vi "DM-Lin Haobo.vi"() -> ()   [LabVIEW 2017]
panel:
  in  "?":T1(tab)=enum."介电频谱测试"
  in  "测试频率4":dbl=1000.0
  in  "测试频率3":dbl=1000.0
  in  "测试频率1":dbl=1000.0
  in  "测试频率2":dbl=1000.0
  in  "变温速率":dbl=2.0
  in  "结束温度":dbl=200.0
  in  "开始温度":dbl=-60.0
  in  "功能选择":u16(ring) items=["Cp-D", "Cp-Q", "Cp-G", "Cp-Rp", "Cs-D", "Cs-Q", "Cs-Rs", "Lp-D", "Lp-Q", "Lp-G", "Lp-Rp", "Lp-Rdc", "Ls-D", "Ls-Q", "Ls-Rs", "Ls-Rdc", "R-X", "Z-thd", "Z-thr", "G-B", "Y-thd", "Y-thr", "Vdc-Idc"]
  in  "低温":bool
  in  "TCC趋势":bool
  out "残差（损耗）":dbl=100000.0
  out "残差（电容）":dbl=3.0
  in  "LT拟合":u16(ring) items=["多项式", "高斯分布"]
  in  "CT拟合":u16(ring) items=["多项式", "高斯分布", "文献的公式"]
  in  "低温 2":bool
  out "TCC(ppm/℃)":dbl
  in  "表格（L）路径：":path=path "C:/Users/Scrooge/Desktop/CL_LT.xls"
  in  "文本（L）路径：":path=path "C:/Users/Scrooge/Desktop/CL_LT.txt"
  out "LT_LT":cluster{dbl[], dbl[]}(graph)={[50.95, 50.95], [0.0151538, 0.0149556]}
  out "CT_LT":cluster{dbl[], dbl[]}(graph)={[50.95, 50.95], [6.54211e-10, 6.56813e-10]}
  in  "表格（R）路径：":path=path "C:/Users/Scrooge/Desktop/CT_RT.xls"
  in  "文本（R）路径：":path=path "C:/Users/Scrooge/Desktop/CT_RT.txt"
  in  "测试时长（s）":dbl
  in  "测试频率（Hz）":dbl
  in  "开始测量":bool
  out "LT_RT":cluster{dbl[], dbl[]}(graph)
  out "CT_RT":cluster{dbl[], dbl[]}(graph)
  out "?":cluster{dbl[], dbl[]}(graph)={[-5.0, -4.5, -4.0, -3.5, -3.0, -2.5, -2.0, -1.5, -1.0, -0.5, 0.0, 0.5, 1.0, 1.5, 2.0, 2.5, 3.0, 3.5, 4.0, 4.5, 5.0, 5.0, 4.5, 4.0], [0.500691, 0.0469761, 0.379431, 0.495874, 0.487151, 0.476265, 0.495886, 0.531751, 0.471661, 0.519222, 0.521993, 0.503018, 0.492567, 0.515073, 0.507819, 0.532721, 0.517626, 0.519501, 0.453623, 0.435659, 0.488314, 0.175289, 0.0581771, 0.0726732]}
  out "?":cluster{dbl[], dbl[]}(graph)={[-5.0, -4.5, -4.0, -3.5, -3.0, -2.5, -2.0, -1.5, -1.0, -0.5, 0.0, 0.5, 1.0, 1.5, 2.0, 2.5, 3.0, 3.5, 4.0, 4.5, 5.0, 5.0, 4.5, 4.0], [-2.02996e-14, -1.53002e-14, -1.24858e-14, -1.27389e-14, -1.22856e-14, -1.3154e-14, -1.26241e-14, -1.25456e-14, -1.26669e-14, -1.291e-14, -1.26131e-14, -1.30559e-14, -1.2444e-14, -1.26388e-14, -1.22714e-14, -1.28488e-14, -1.30514e-14, -1.28353e-14, -1.3487e-14, -1.35321e-14, -1.2498e-14, -1.39281e-14, -1.68177e-14, -1.62818e-14]}
  in  "文本（BI）路径：":path=path "C:/Users/shipeng/Desktop/BIAS Dielectric measurement Log"
  in  "起始偏压":dbl[][](array[numeric])=[[-5.0, 5.0, 21.0], [5.0, -5.0, 21.0], [-5.0, 0.0, 10.0]]
  in  "偏压":bool
  in  "表格（BI）路径：":path=path "C:/Users/shipeng/Desktop/BIAS Dielectric measurement Log"
  in  "时间间隔(s)":dbl=2.0
  in  "开始频率":dbl[](array[numeric])=[10.0, 10000.0, 100.0]
  in  "频谱":bool
  in  "Scanning Mode":u16(ring)=1 items=["Linear", "Log"]
  in  "文本（SP）路径：":path=path "C:/Users/Scrooge/Desktop/SP.txt"
  out "?":cluster{dbl[], dbl[]}(graph)={[20.0, 22.675383571384522, 25.708651005470756, 29.147676132595485, 33.04673682605462, 37.46737166566934, 42.47935119653383, 48.16177911224783, 54.604340742525736, 61.90871854996752, 70.19019697667008, 79.57948196985141, 90.22476390392299, 102.29405645795312, 115.97784836284757, 131.49210987057194, 149.08170139629277, 169.0242381317775, 191.63447162495464, 217.26925747977248, 246.33318758118733, 279.28497573826183, 316.6446975294954, 359.00199861631705, 407.0254010759322, 461.4728546346695, 523.2036993311451, 593.1922284150527, 672.5430655437831, 762.5085989740041, 864.5087479107281, 980.1533729846564, 1111.2676845606702, 1259.921049894877, 1428.4596538013916, 1619.5435283096847, 1836.1885357487772, 2081.8139678741213, 2360.296512290584, 2676.0314379195047, 3034.0019651954212, 3439.8579158570305, 3900.0048836560754, 4421.705333358719, 5013.193223677282, 5683.803963217401, 6444.121750525505, 7306.146623693386, 8283.483856051174, 9391.558687166586, 10647.85977823354, 12072.215234288142, 13687.105549689764, 15518.01841606206, 17593.850992600805, 19947.365987750378, 22615.70875055146, 25640.99353287359, 29070.968175464932, 32959.76770850899, 37368.76876070874, 42367.55826197211, 48035.031728659946, 54460.63846554949, 61745.793337441646, 70005.47739229642, 79370.05259841043, 89987.31933749607, 102024.84912691955, 115672.62938827681, 131146.0620044891, 148689.36299141843, 168579.41694076196, 191130.14706860675, 216697.46984178963, 245684.9123805555, 278549.9812965547, 315811.3834850681, 358057.21283667657, 405954.2320786253, 460258.39624048397, 521826.78383516293, 591631.1240642137, 670773.1335462716, 760501.904627062, 862233.6197093561, 977573.9027526472, 1108343.1607145814, 1256605.3148961905, 1424700.3756555775, 1615281.374614292, 1831356.2372546163, 2076335.256779795, 2354084.9185135514, 2668988.924345313, 3026017.3803653475, 3430805.2396730217, 3889741.2384150787, 4410068.728724708, 5000000.000000043], [106196000.0, 92409900.0, 81785700.0, 73412700.0, 64489800.0, 57461600.0, 50488800.0, 43921400.0, 38435000.0, 34246700.0, 30339600.0, 26557900.0, 23615000.0, 20839100.0, 18326800.0, 16247600.0, 14299300.0, 12599900.0, 11076900.0, 9796620.0, 8640500.0, 7619490.0, 6707090.0, 5922820.0, 5224210.0, 4612170.0, 4065330.0, 3585910.0, 3159420.0, 2786990.0, 2458510.0, 2169980.0, 1914220.0, 1687870.0, 1489290.0, 1312820.0, 1158360.0, 1021520.0, 901184.0, 794774.0, 700688.0, 618030.0, 545151.0, 480780.0, 424064.0, 374013.0, 329921.0, 290997.0, 256820.0, 226380.0, 199671.0, 176131.0, 155324.0, 137024.0, 120843.0, 106591.0, 94025.6, 82911.0, 73148.6, 64507.3, 56898.9, 50186.7, 44265.8, 39042.2, 34436.3, 30373.6, 26787.8, 23625.0, 20844.2, 18379.7, 16209.0, 14295.6, 12607.4, 11117.7, 9803.59, 8652.08, 7630.04, 6728.0, 5932.48, 5229.76, 4609.8, 4062.43, 3579.4, 3163.33, 2787.36, 2455.53, 2162.54, 1904.44, 1676.44, 1474.35, 1299.56, 1140.07, 995.777, 823.897, 705.8, 596.582, 494.824, 397.785, 377.206, 304.016]}
  out "?":cluster{dbl[], dbl[]}(graph)={[20.0, 22.675383571384522, 25.708651005470756, 29.147676132595485, 33.04673682605462, 37.46737166566934, 42.47935119653383, 48.16177911224783, 54.604340742525736, 61.90871854996752, 70.19019697667008, 79.57948196985141, 90.22476390392299, 102.29405645795312, 115.97784836284757, 131.49210987057194, 149.08170139629277, 169.0242381317775, 191.63447162495464, 217.26925747977248, 246.33318758118733, 279.28497573826183, 316.6446975294954, 359.00199861631705, 407.0254010759322, 461.4728546346695, 523.2036993311451, 593.1922284150527, 672.5430655437831, 762.5085989740041, 864.5087479107281, 980.1533729846564, 1111.2676845606702, 1259.921049894877, 1428.4596538013916, 1619.5435283096847, 1836.1885357487772, 2081.8139678741213, 2360.296512290584, 2676.0314379195047, 3034.0019651954212, 3439.8579158570305, 3900.0048836560754, 4421.705333358719, 5013.193223677282, 5683.803963217401, 6444.121750525505, 7306.146623693386, 8283.483856051174, 9391.558687166586, 10647.85977823354, 12072.215234288142, 13687.105549689764, 15518.01841606206, 17593.850992600805, 19947.365987750378, 22615.70875055146, 25640.99353287359, 29070.968175464932, 32959.76770850899, 37368.76876070874, 42367.55826197211, 48035.031728659946, 54460.63846554949, 61745.793337441646, 70005.47739229642, 79370.05259841043, 89987.31933749607, 102024.84912691955, 115672.62938827681, 131146.0620044891, 148689.36299141843, 168579.41694076196, 191130.14706860675, 216697.46984178963, 245684.9123805555, 278549.9812965547, 315811.3834850681, 358057.21283667657, 405954.2320786253, 460258.39624048397, 521826.78383516293, 591631.1240642137, 670773.1335462716, 760501.904627062, 862233.6197093561, 977573.9027526472, 1108343.1607145814, 1256605.3148961905, 1424700.3756555775, 1615281.374614292, 1831356.2372546163, 2076335.256779795, 2354084.9185135514, 2668988.924345313, 3026017.3803653475, 3430805.2396730217, 3889741.2384150787, 4410068.728724708, 5000000.000000043], [106196000.0, 92409900.0, 81785700.0, 73412700.0, 64489800.0, 57461600.0, 50488800.0, 43921400.0, 38435000.0, 34246700.0, 30339600.0, 26557900.0, 23615000.0, 20839100.0, 18326800.0, 16247600.0, 14299300.0, 12599900.0, 11076900.0, 9796620.0, 8640500.0, 7619490.0, 6707090.0, 5922820.0, 5224210.0, 4612170.0, 4065330.0, 3585910.0, 3159420.0, 2786990.0, 2458510.0, 2169980.0, 1914220.0, 1687870.0, 1489290.0, 1312820.0, 1158360.0, 1021520.0, 901184.0, 794774.0, 700688.0, 618030.0, 545151.0, 480780.0, 424064.0, 374013.0, 329921.0, 290997.0, 256820.0, 226380.0, 199671.0, 176131.0, 155324.0, 137024.0, 120843.0, 106591.0, 94025.6, 82911.0, 73148.6, 64507.3, 56898.9, 50186.7, 44265.8, 39042.2, 34436.3, 30373.6, 26787.8, 23625.0, 20844.2, 18379.7, 16209.0, 14295.6, 12607.4, 11117.7, 9803.59, 8652.08, 7630.04, 6728.0, 5932.48, 5229.76, 4609.8, 4062.43, 3579.4, 3163.33, 2787.36, 2455.53, 2162.54, 1904.44, 1676.44, 1474.35, 1299.56, 1140.07, 995.777, 823.897, 705.8, 596.582, 494.824, 397.785, 377.206, 304.016]}
  in  "表格（SP）路径：":path=path "C:/Users/Scrooge/Desktop/SP.xls"
  in  "使用6517B":bool
  in  "样本厚度(mm)":dbl
  in  "样本直径(mm)":dbl
  in  "电压(V)":dbl
  in  "测试时间":dbl
  in  "绝缘":bool
  out "?":cluster{dbl[], dbl[]}(graph)={[0.201, 1.192, 2.172, 3.151, 4.129, 5.107, 6.086, 7.064, 8.042, 9.021, 10.0, 10.978, 11.957, 12.935, 13.913, 14.891, 15.87, 16.849, 17.827, 18.807, 19.789, 20.767, 21.746, 22.724, 23.702, 24.68, 25.659, 26.637, 27.616, 28.595, 29.558, 30.536, 31.514, 32.493, 33.472, 34.45, 35.43, 36.408, 37.386, 38.365, 39.344, 40.339], [-1675.86, -1675.85, -1676.0, -1676.13, -1676.17, -1676.27, -1677.48, -1675.99, -1676.43, -1681.46, -1676.29, -1676.08, -1676.1, -1676.02, -1675.83, -1675.8, -1675.82, -1675.56, -1675.6, -1675.32, -1675.21, -1674.89, -1674.7, -1674.46, -1673.99, -1673.55, -1673.08, -1672.36, -1671.64, -1670.87, -1670.26, -1669.55, -1668.7, -1667.65, -1666.77, -1665.8, -1664.61, -1663.41, -1662.55, -1661.04, -1659.56, -1657.68]}
  out "?":cluster{dbl[], dbl[]}(graph)={[0.201, 1.192, 2.172, 3.151, 4.129, 5.107, 6.086, 7.064, 8.042, 9.021, 10.0, 10.978, 11.957, 12.935, 13.913, 14.891, 15.87, 16.849, 17.827, 18.807, 19.789, 20.767, 21.746, 22.724, 23.702, 24.68, 25.659, 26.637, 27.616, 28.595, 29.558, 30.536, 31.514, 32.493, 33.472, 34.45, 35.43, 36.408, 37.386, 38.365, 39.344, 40.339], [9665.96, 9670.54, 9661.83, 9662.16, 9663.16, 9703.15, 9737.63, 9698.46, 9692.46, 9806.7, 9560.83, 9481.19, 9418.37, 9320.17, 9268.16, 9226.14, 9160.9, 9088.06, 9034.83, 8929.32, 8815.93, 8688.35, 8579.32, 8438.3, 8233.36, 8027.73, 7834.66, 7575.86, 7313.56, 7056.58, 6882.85, 6681.73, 6437.13, 6185.99, 5948.9, 5748.35, 5507.66, 5280.44, 5128.46, 4857.69, 4620.19, 4342.91]}
  in  "文本（IN）路径：":path=path "C:/Users/Scrooge/Desktop/IN.txt"
  in  "表格（IN）路径：":path=path "C:/Users/Scrooge/Desktop/IN.xls"
  out "样品温度":dbl
  out "设定温度":dbl
  out "炉丝温度":dbl
  in  "测试温度":dbl
  out "当前频率":dbl
  in  "开始测量":bool
  out "?":cluster{dbl[], dbl[]}(graph)={[4.76578, 4.95183, 5.2639, 5.45631, 5.68923, 5.96482, 6.29877, 6.6422, 6.96399, 7.34085, 7.76822, 8.17855, 8.63274, 9.15865, 9.79553, 10.5502, 11.0706, 11.9952, 12.9319, 13.9265, 15.0197, 16.3568, 17.7532, 19.3246, 21.0927, 23.0242, 25.0623, 27.5307, 29.9738, 33.2177, 36.5272, 40.3473, 44.6699, 49.3322, 54.7469, 60.6627, 67.4071, 74.9786, 83.5253, 93.1379, 104.03, 116.389, 130.429, 145.987, 163.909, 183.98, 206.64, 232.188, 258.147, 291.919, 335.859, 374.84, 414.539, 465.991, 532.048, 602.949, 689.134, 773.249, 870.102, 985.903, 1123.13, 1275.36, 1451.73, 1641.81, 1865.44, 2115.4, 2399.17, 2720.93, 3089.67, 3508.29, 3980.83, 4515.29, 5118.64, 5799.71, 6605.19, 7472.24, 8449.86, 9551.85, 10779.4, 12163.7, 13702.2, 15433.1, 17391.2, 19544.4, 21947.6, 24613.1, 27562.8, 30840.7, 34475.5, 38529.5, 42968.4, 47826.9, 53184.8, 59163.2, 65651.7, 72759.1, 80688.8, 89228.1, 98569.2, 109036.0, 119923.0, 132208.0, 145083.0, 160265.0, 175774.0, 193159.0, 211401.0, 233068.0, 252305.0, 278064.0, 302611.0, 331752.0, 363430.0, 397628.0, 432832.0, 469048.0, 511668.0, 554491.0, 605253.0, 655000.0, 713841.0, 767324.0, 831011.0, 905837.0, 971237.0, 1047330.0, 1135590.0, 1242550.0, 1324860.0, 1419260.0, 1528060.0, 1657260.0, 1657060.0, 1657050.0, 1656970.0], [-83.8388, -94.0695, -105.065, -116.633, -129.293, -142.98, -157.704, -173.594, -190.768, -209.471, -229.697, -251.716, -275.643, -301.645, -329.901, -360.642, -393.025, -429.595, -469.363, -512.712, -559.92, -611.338, -667.345, -728.401, -794.926, -867.436, -946.529, -1032.74, -1127.27, -1229.64, -1341.14, -1462.94, -1595.66, -1740.3, -1897.85, -2069.31, -2256.7, -2460.9, -2683.52, -2926.12, -3190.55, -3478.51, -3792.28, -4134.43, -4507.09, -4913.34, -5355.9, -5837.88, -6361.18, -6940.5, -7557.26, -8227.75, -8966.19, -9776.49, -10656.2, -11603.4, -12634.8, -13758.9, -14987.4, -16326.3, -17778.6, -19343.5, -21058.8, -22912.4, -24935.1, -27125.7, -29507.3, -32090.3, -34889.3, -37930.7, -41217.4, -44779.7, -48622.7, -52802.5, -57377.3, -62244.1, -67524.9, -73242.8, -79372.7, -86027.9, -93155.5, -100863.0, -109184.0, -118105.0, -127741.0, -138062.0, -149118.0, -160966.0, -173746.0, -187598.0, -202286.0, -217928.0, -234691.0, -252890.0, -272113.0, -292631.0, -314916.0, -338309.0, -363290.0, -390625.0, -418327.0, -449446.0, -481377.0, -517085.0, -552683.0, -591702.0, -631650.0, -677951.0, -720582.0, -773764.0, -824284.0, -882606.0, -943903.0, -1007950.0, -1073950.0, -1140070.0, -1216170.0, -1291290.0, -1378160.0, -1461580.0, -1558420.0, -1642670.0, -1743870.0, -1859760.0, -1958990.0, -2071380.0, -2200810.0, -2350980.0, -2464640.0, -2593280.0, -2739320.0, -2906600.0, -2906310.0, -2905990.0, -2905750.0]}
  in  "表格（CC）路径：":path=path "C:/Users/Scrooge/Desktop/CC.xls"
  in  "文本（CC）路径：":path=path "C:/Users/Scrooge/Desktop/CC.txt"
  in  "开始频率":dbl[](array[numeric])=[20.0, 5000000.0, 100.0]
  in  "扫描模式":u16(ring)=1 items=["Linear", "Log"]
  in  "极化开始":bool
  out "剩余时间":dbl
  out "极化状态":bool
  out "当前温度":dbl
  in  "结束冷却":bool
  in  "结束温度（℃）":dbl
  in  "变温速率（℃/min）":dbl
  in  "极化时间":dbl
  in  "极化电压（V）":dbl
  in  "极化温度（℃）":dbl
  out "当前去极化电流":dbl
  in  "文本（TSDC）路径：":path=path "C:/Users/Scrooge/Desktop/TSDC.txt"
  out "?":cluster{dbl[], dbl[]}(graph)
  in  "温度":bool
  in  "变温速率1":dbl=3.0
  in  "目标温度":dbl=255.0
  out "TE":cluster{dbl[], dbl[]}(graph)={[0.0, 2.0, 4.0, 6.001, 8.001, 10.001, 12.001, 14.002, 16.002, 18.002, 20.003, 22.003, 24.003, 26.003, 28.003, 30.003, 32.003, 34.003, 36.003, 38.003, 40.003, 42.004, 44.004, 46.004, 48.005, 50.006, 52.006, 54.006, 56.006, 58.007, 60.007, 62.007, 64.007, 66.007, 68.007, 70.007, 72.007, 74.008, 76.008, 78.008, 80.008, 82.008, 84.008, 86.008, 88.008, 90.008, 92.008, 94.008, 96.008, 98.008, 100.009, 102.01, 104.01, 106.01, 108.01, 110.01, 112.01, 114.01, 116.01, 118.01, 120.01, 122.01, 124.011, 126.012, 128.012, 130.013, 132.013, 134.014, 136.014, 138.014, 140.014, 142.014, 144.014, 146.014, 148.014, 150.014, 152.015, 154.015, 156.016, 158.016, 160.016, 162.016, 164.016, 166.016, 168.016, 170.016, 172.017, 174.017, 176.018, 178.018, 180.019, 182.019, 184.019, 186.019, 188.02, 190.02, 192.02, 194.02, 196.021, 198.021, 200.021, 202.022, 204.022, 206.022, 208.022, 210.023, 212.023, 214.023, 216.023, 218.023, 220.023, 222.024, 224.025, 226.025, 228.026, 230.026, 232.026, 234.026, 236.026, 238.026, 240.026, 242.026, 244.027, 246.028, 248.028, 250.028, 252.028, 254.028, 256.028, 258.028, 260.028, 262.028, 264.028, 266.028, 268.028, 270.029, 272.029, 274.029, 276.029, 278.029, 280.029, 282.03, 284.03, 286.03, 288.031, 290.031, 292.031, 294.031, 296.031, 298.031, 300.031, 302.032, 304.032, 306.032, 308.032, 310.032, 312.032, 314.032, 316.615, 318.616, 320.616, 322.616, 324.616, 326.616, 328.616, 330.616, 332.616, 334.617, 336.617, 338.617, 340.617, 342.617, 344.617, 346.617, 348.617, 350.617, 352.617, 354.618, 356.618, 358.618, 360.618, 362.618, 364.619, 366.619, 368.619, 370.62, 372.62, 374.62, 376.621, 378.621, 380.622, 382.622, 384.622, 386.622, 388.622, 390.623, 392.623, 394.623, 396.623, 398.623, 400.624, 402.624, 404.624, 406.624, 408.624, 410.625, 412.625, 414.625, 416.625, 418.625, 420.625, 422.625, 424.626, 426.626, 428.626, 430.627, 432.627, 434.627, 436.627, 438.628, 440.628, 442.628, 444.628, 446.628, 448.628, 450.628, 452.628, 454.629, 456.629, 458.63, 460.63, 462.63, 464.63, 466.63, 468.63, 470.63, 472.63, 474.63, 476.63, 478.631, 480.631, 482.632, 484.632, 486.632, 488.632, 490.632, 492.633, 494.633, 496.633, 498.633, 500.633, 502.633, 504.633, 506.633, 508.633, 510.633, 512.633, 514.633, 516.633, 518.633, 520.633, 522.633, 524.633, 526.633, 528.633, 530.634, 532.634, 534.634, 536.634, 538.634, 540.634, 542.635, 544.635, 546.635, 548.635, 550.635, 552.635, 554.636, 581.094, 583.094, 585.095, 587.095, 589.095, 591.095, 593.096, 595.097, 597.097, 599.097, 601.097, 603.097, 605.097, 607.097, 609.097, 611.098, 613.099, 615.099, 617.099, 621.973, 623.973, 625.973, 627.973, 629.973, 631.973, 633.973, 635.973, 637.973, 639.973, 641.973, 643.974, 648.231, 650.231, 652.231, 654.231, 656.231, 658.231, 660.231, 662.231, 664.231, 666.231, 668.231], [50.0, 50.0, 49.96, 49.910000000000004, 49.84, 49.77, 49.72, 49.68, 49.63, 49.47, 49.46, 49.51, 49.57, 49.64, 49.77, 49.85, 49.77, 49.800000000000004, 49.88, 50.0, 50.13, 50.29, 50.370000000000005, 50.5, 50.620000000000005, 50.74, 50.92, 50.84, 50.910000000000004, 50.980000000000004, 51.06, 51.14, 51.31, 51.43, 51.550000000000004, 51.68, 51.76, 51.88, 51.83, 51.910000000000004, 51.99, 52.120000000000005, 52.2, 52.28, 52.36, 52.480000000000004, 52.61, 52.78, 52.86, 52.75, 52.81, 52.88, 52.96, 53.09, 53.21, 53.33, 53.42, 53.54, 53.620000000000005, 53.71, 53.620000000000005, 53.65, 53.78, 53.86, 53.93, 54.02, 54.1, 54.18, 54.27, 54.43, 54.550000000000004, 54.46, 54.54, 54.620000000000005, 54.75, 54.88, 55.04, 55.21, 55.33, 55.45, 55.58, 55.75, 55.69, 55.78, 55.86, 55.980000000000004, 56.07, 56.24, 56.36, 56.49, 56.61, 56.74, 56.78, 56.79, 56.88, 57.0, 57.08, 57.17, 57.25, 57.410000000000004, 57.54, 57.660000000000004, 57.78, 57.870000000000005, 57.78, 57.86, 57.99, 58.11, 58.230000000000004, 58.31, 58.44, 58.52, 58.69, 58.85, 58.89, 58.85, 58.93, 59.050000000000004, 59.18, 59.34, 59.42, 59.550000000000004, 59.67, 59.79, 59.96, 59.99, 60.01, 60.09, 60.18, 60.300000000000004, 60.47, 60.59, 60.71, 60.84, 60.96, 61.08, 61.14, 61.13, 61.21, 61.34, 61.42, 61.5, 61.67, 61.79, 61.910000000000004, 62.04, 62.160000000000004, 62.190000000000005, 62.17, 62.29, 62.410000000000004, 62.5, 62.620000000000005, 62.7, 62.83, 62.96, 63.120000000000005, 63.13, 63.120000000000005, 63.24, 63.32, 63.52, 63.65, 63.77, 63.85, 63.980000000000004, 64.06, 64.26, 64.29, 64.29, 64.37, 64.5, 64.62, 64.78, 64.91, 65.03, 65.15, 65.28, 65.36, 65.48, 65.49, 65.57000000000001, 65.65, 65.78, 65.86, 66.03, 66.16, 66.28, 66.36, 66.53, 66.44, 66.48, 66.61, 66.73, 66.85, 66.94, 67.02, 67.14, 67.31, 67.43, 67.55, 67.5, 67.55, 67.63, 67.8, 67.92, 68.0, 68.17, 68.25, 68.37, 68.55, 68.67, 68.65, 68.65, 68.73, 68.85000000000001, 69.02, 69.18, 69.3, 69.43, 69.55, 69.67, 69.84, 69.8, 69.84, 69.93, 70.01, 70.13, 70.3, 70.42, 70.54, 70.67, 70.79, 70.91, 70.87, 70.95, 71.03, 71.12, 71.2, 71.32000000000001, 71.45, 71.61, 71.73, 71.86, 71.98, 71.88, 71.94, 72.10000000000001, 72.18, 72.31, 72.43, 72.5, 72.67, 72.83, 72.95, 73.08, 73.05, 73.07000000000001, 73.16, 73.29, 73.41, 73.54, 73.7, 73.82000000000001, 73.91, 74.08, 74.2, 74.16, 74.23, 74.29, 74.42, 74.55, 74.67, 74.8, 74.92, 75.04, 75.17, 76.37, 76.4, 76.53, 76.65, 76.73, 76.82000000000001, 76.98, 77.15, 77.28, 77.4, 77.47, 77.41, 77.49, 77.62, 77.75, 77.87, 77.99, 78.08, 78.2, 78.56, 78.48, 78.51, 78.56, 78.63, 78.71000000000001, 78.79, 78.92, 79.04, 79.12, 79.25, 79.33, 79.25, 79.26, 79.28, 79.33, 79.35000000000001, 79.42, 79.47, 79.52, 79.58, 79.69, 79.53, 79.52]} caption="1"
  in  "远程模式":bool
  out "错误输出":cluster{"状态":bool, "代码":i32, "源":string}={"状态"=FALSE, "代码"=-1950679034, "源"="DM-Lin Haobo.vi中的共享变量<APPEND>\n读取以下共享变量时发生该错误或警告：\n\\\\我的电脑\\Input\\Start_LT\n\\\\10.21.14.98\\Input\\Start_LT"}
  in  "error in (no error)":errorcluster caption="错误输入（无错误）"
  in  "电阻计地址":refnum<visa-resource-name>
  in  "低温地址":refnum<visa-resource-name>
  in  "高温地址 1":refnum<visa-resource-name> caption="高温地址1"
  in  "高温地址 2":refnum<visa-resource-name> caption="高温地址2"
  in  "电容计地址":refnum<visa-resource-name>
  # "参数1-温度"
  # "参数2-温度/TCC"
  # "电容-时间"
  # "损耗-时间"
  # "结束偏压"
  # "步长"
  # "结束频率"
  # "步数"
  # "基本功能"
  # "K6517B功能"
  # "电阻值（TH2826）-时间\n电阻率（K6517B）-时间"
  # "电抗（TH2826）-时间\n电流（K6517B）-时间"
  # "Z'-Z''(R-X)"
  # "操作步骤：\n1.输入数据保存路径\n2.设置极化温度、极化电压、极化时间\n3.点击“极化开始”按钮，等待温度达到极化温度\n4.当极化温度达到设定温度后观察“极化状态”指示灯\n5.若“极化状态”指示灯亮起，则意味着极化电压已正常启动\n6.极化电压启动后观察“剩余时间”，当其为0时极化结束\n7.极化结束后请尽快开启液氮冷却样品\n8.要开始测电流请先在“结束温度”输入框内填入测量结束温度\n9.按下“结束冷却”按钮，极化电压将关闭，TSDC测量开始\n注意：\n1.“变温速率”=极化前升温速=极化后降温速=测电流升温速\n2.开始测电流的三个条件：\n2.1.“结束冷却”按钮被按下\n2.2.“当前温度”低于-20（摄氏度）\n2.3.“剩余时间”为0"
  # "TSDC-温度"
  # "温度-时间"
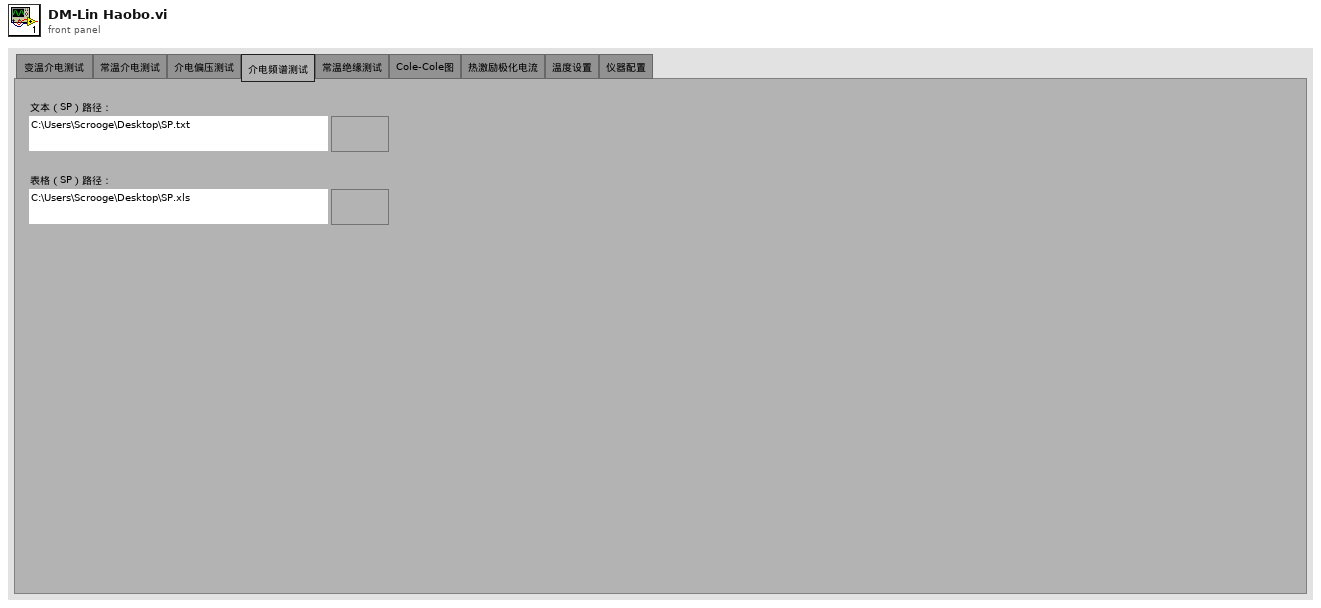
[diagram p1: front panel]
types:
  T1 = enum32{"变温介电测试 ", "常温介电测试", "介电偏压测试", "介电频谱测试", "常温绝缘测试", "Cole-Cole图", "热激励极化电流", "温度设置", "仪器配置"}
  T2 = cluster{"测试频率1":dbl, "测试频率2":dbl, "测试频率3":dbl, "测试频率4":dbl}
  T3 = cluster{"CT_LT":cluster{dbl[], dbl[]}, "LT_LT":cluster{dbl[], dbl[]}}
  T4 = cluster{"电容计地址":refnum<visa-resource-name>, "高温地址 1":refnum<visa-resource-name>, "高温地址 2":refnum<visa-resource-name>}
  T5 = cluster{"开始温度":dbl, "变温速率":dbl, "结束温度":dbl, cluster{"测试频率1":dbl, "测试频率2":dbl, "测试频率3":dbl, "测试频率4":dbl}}
  T6 = cluster{"电容计地址":refnum<visa-resource-name>, "低温地址":refnum<visa-resource-name>}
  T7 = cluster{"电阻计地址":refnum<visa-resource-name>, "电容计地址":refnum<visa-resource-name>, "低温地址":refnum<visa-resource-name>, "高温地址 2":refnum<visa-resource-name>}
  T8 = cluster{"电压(V)":dbl, "样本直径(mm)":dbl, "样本厚度(mm)":dbl}
  T9 = cluster{"Ctrl Reference":refnum<vi>, "当前频率":refnum<vi>, "炉丝温度":refnum<vi>, "设定温度":refnum<vi>, "样品温度":refnum<vi>}
  T10 = cluster{"电阻计地址":refnum<visa-resource-name>, "高温地址 1":refnum<visa-resource-name>, "高温地址 2":refnum<visa-resource-name>}
  T11 = cluster{"变温速率（℃/min）":dbl, "极化温度（℃）":dbl, "极化电压（V）":dbl, "极化时间":dbl}
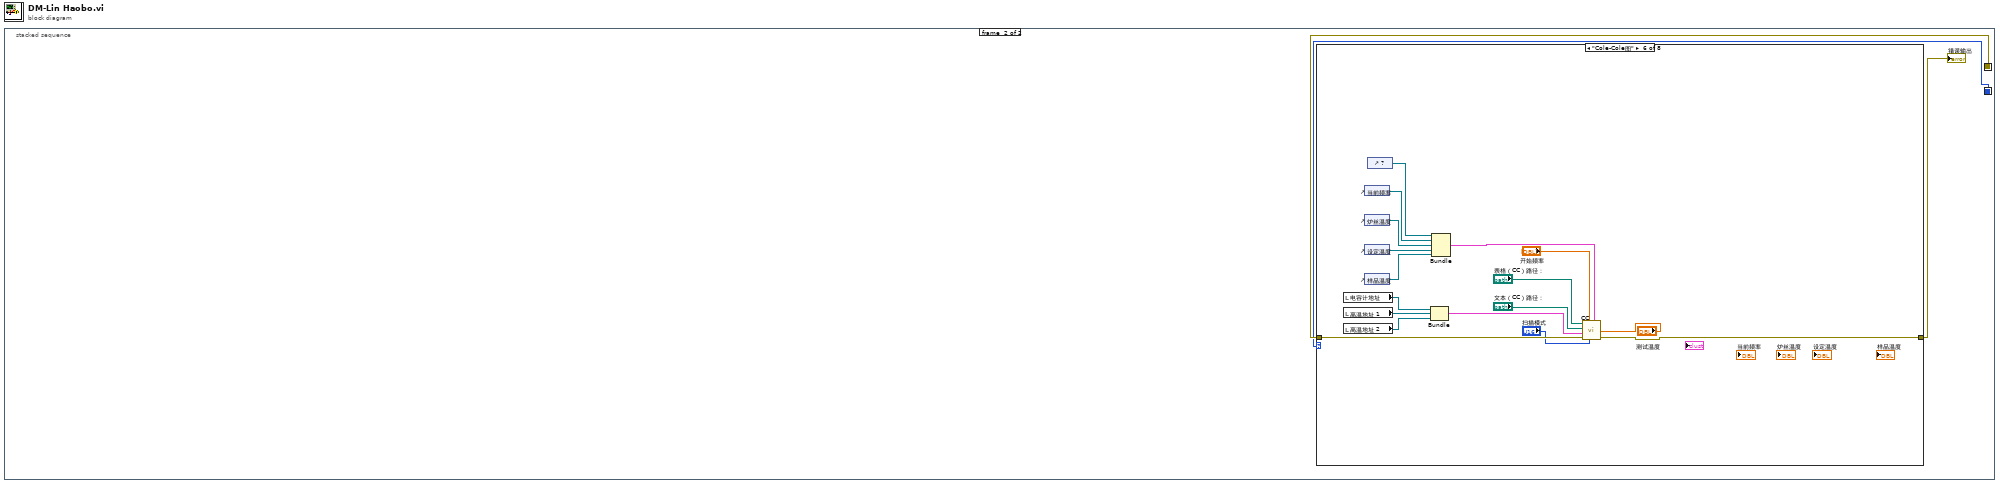
[diagram p0: block diagram]
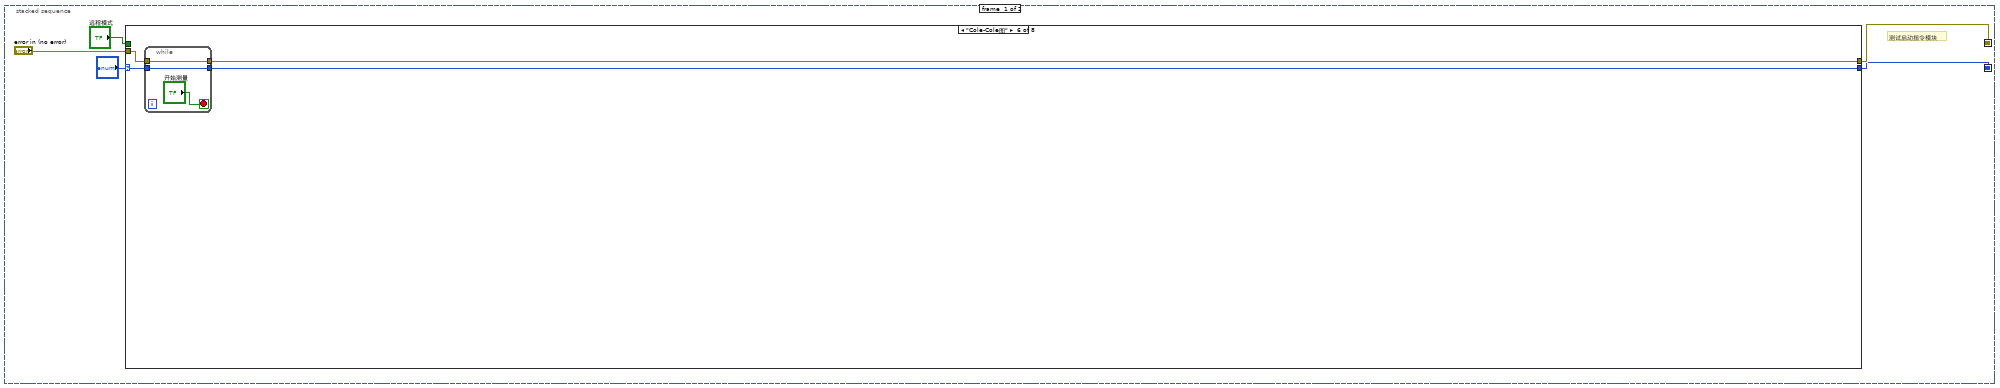
[diagram p2: hidden frame]
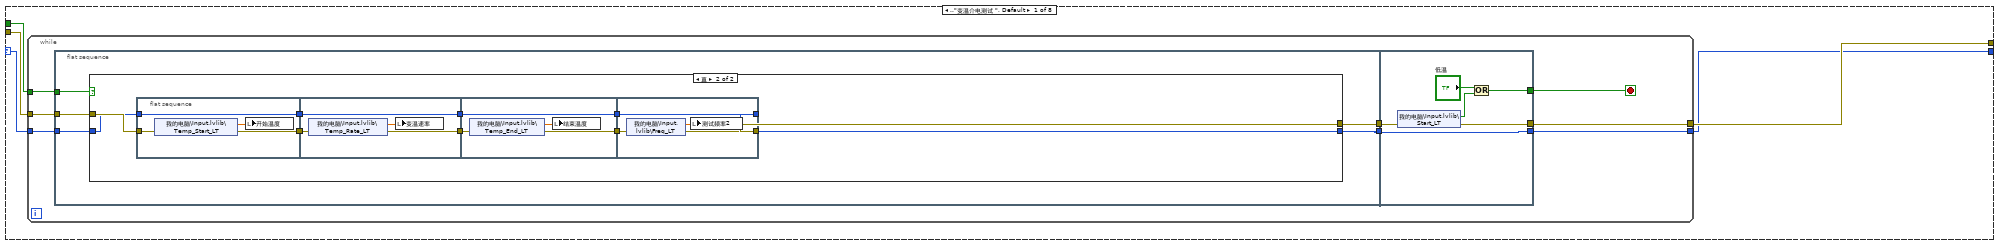
[diagram p3: hidden frame]
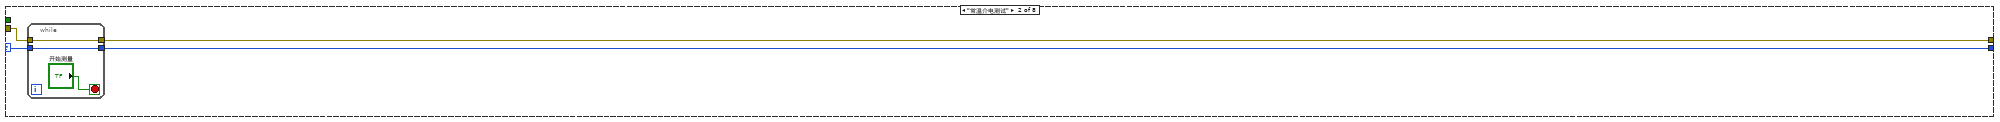
[diagram p5: hidden frame]
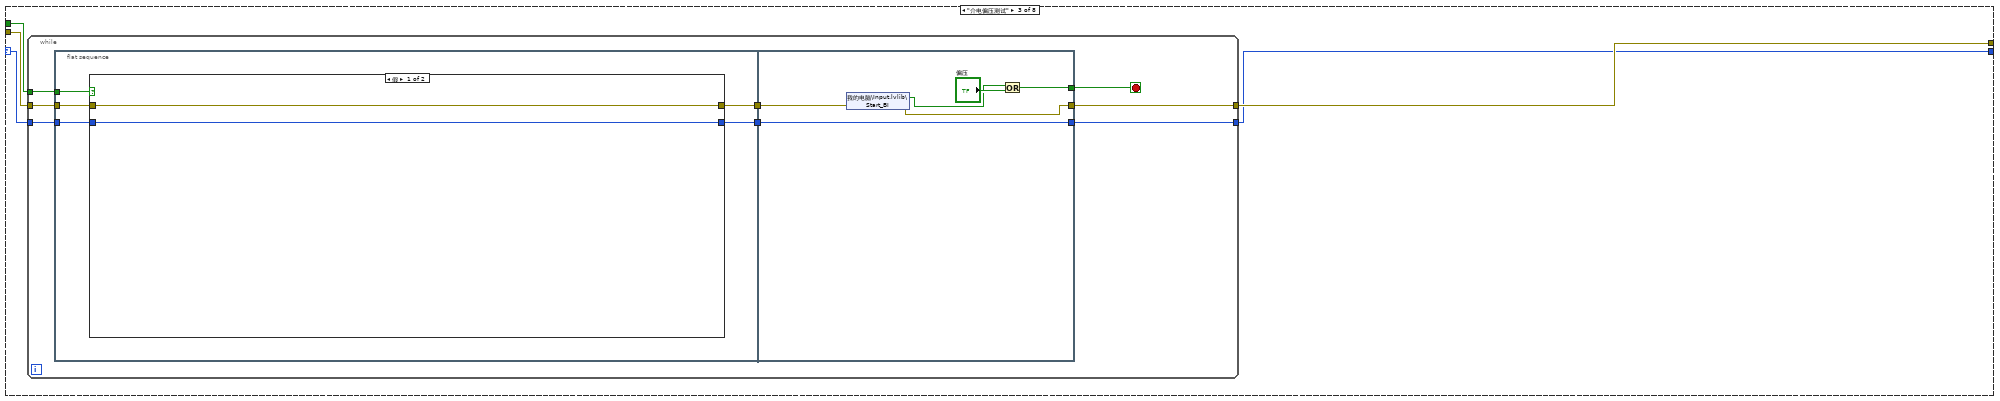
[diagram p6: hidden frame]
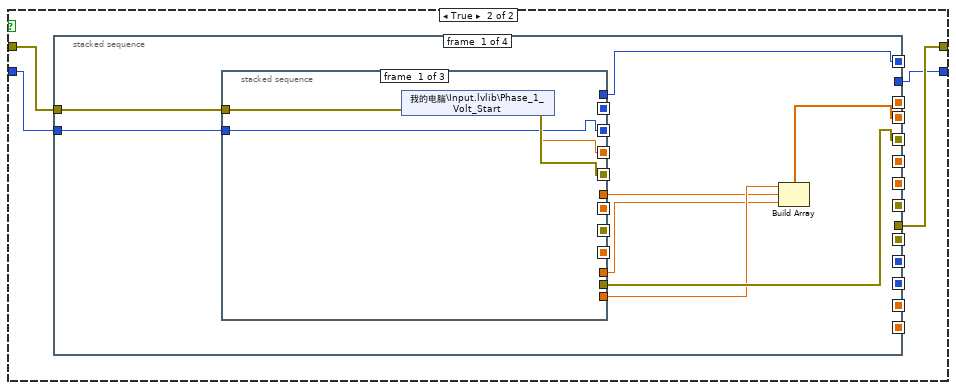
[diagram p7: hidden frame]
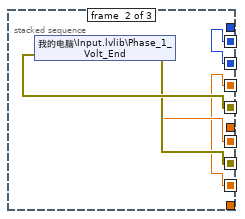
[diagram p8: hidden frame]
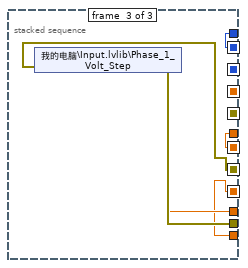
[diagram p9: hidden frame]
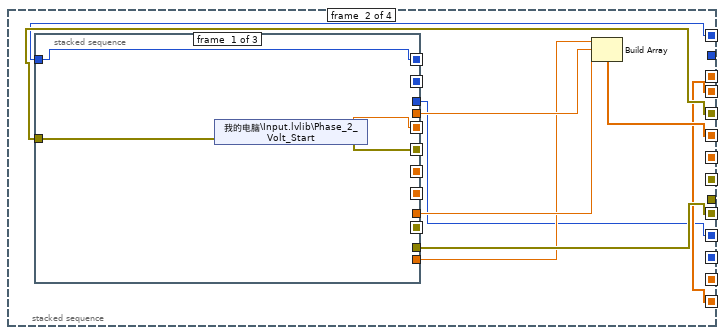
[diagram p10: hidden frame]
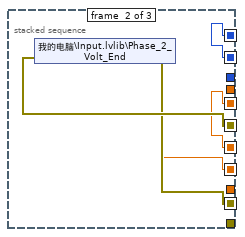
[diagram p11: hidden frame]
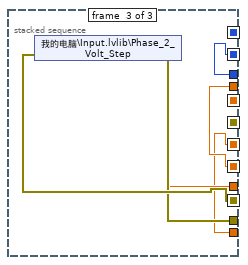
[diagram p12: hidden frame]
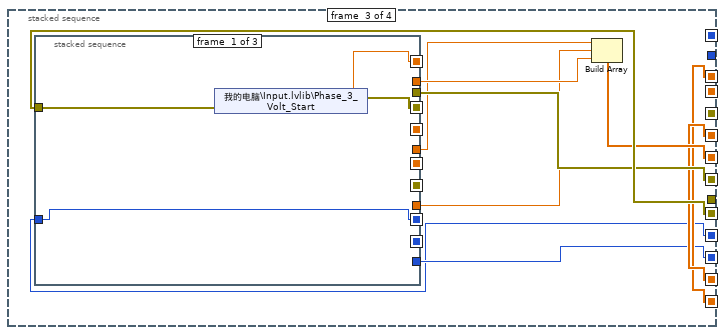
[diagram p13: hidden frame]
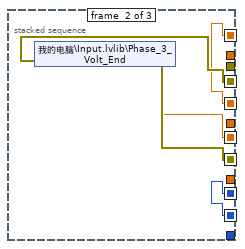
[diagram p14: hidden frame]
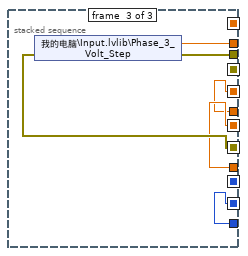
[diagram p15: hidden frame]
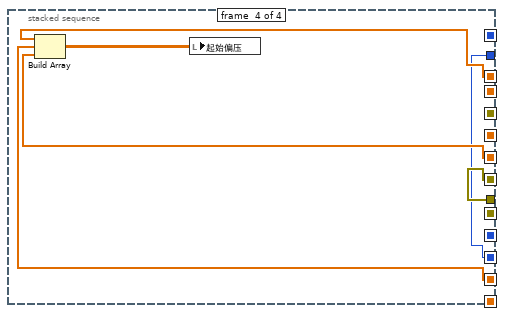
[diagram p16: hidden frame]
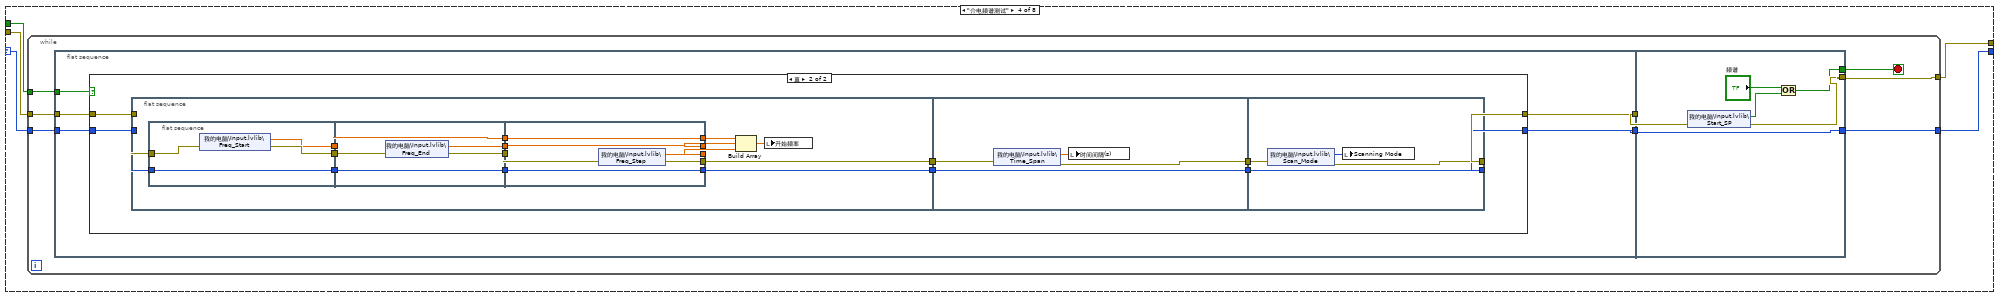
[diagram p17: hidden frame]
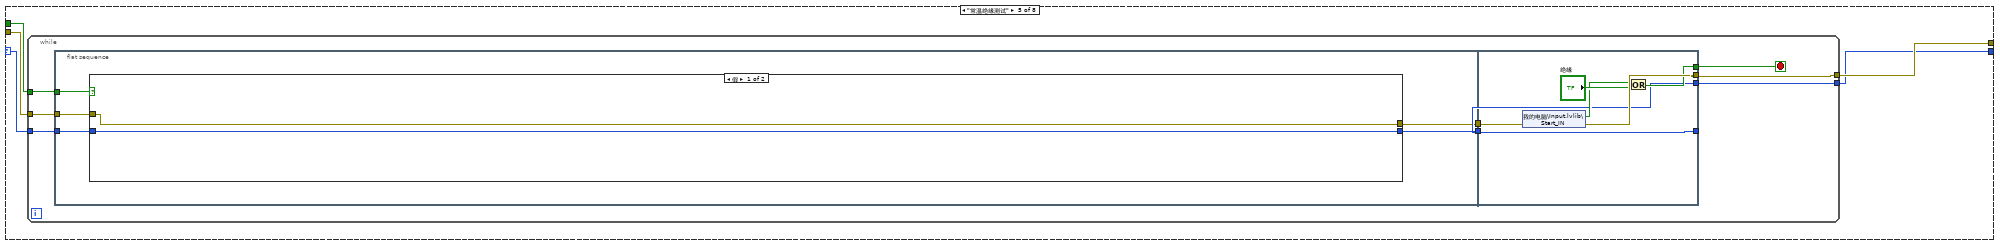
[diagram p19: hidden frame]
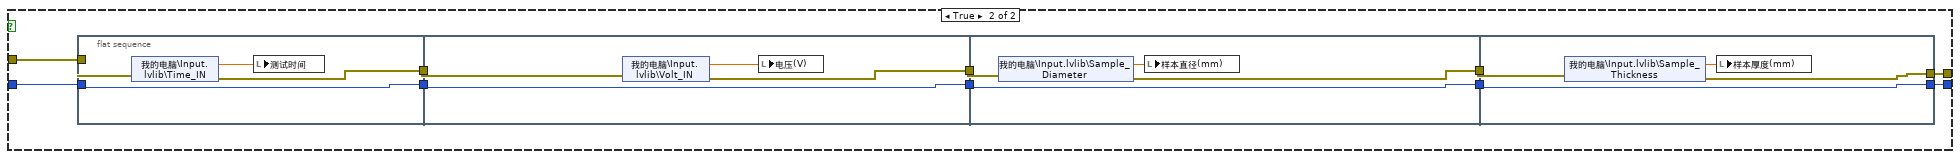
[diagram p20: hidden frame]
diagram:
  n1 = stacked-sequence {
    seq-local: [w1 _] -> [_ w351]
    seq-local: [w5 _] -> [_ w353]
    frame #0 {
      # "测试启动指令模块"
      n2 = case shown="\"Cole-Cole图\"" "?" {
        selector: "?" -> [w6 w59 w66 w173 w246 w300 w305 w312]
        tunnel: [w9 w61 w67 w175 w247 w297 w306 w313] -> w5
        tunnel: "error in (no error)" -> [w10 w60 w69 w177 w249 w298 w307 w315]
        tunnel: "远程模式" -> [w8 _ w68 w176 w248 _ _ w314]
        tunnel: [w7 w58 w65 w174 w245 w299 w304 w311] -> w1
        frame .."变温介电测试 ", Default {
          n3 = while {
            tunnel: w10 -> [w18]
            tunnel: [w17] -> w9
            tunnel: w8 -> [w14]
            tunnel: [w13] -> w7
            tunnel: w6 -> [w11]
            stop <- w16 stop-if-true
            n4 = flat-sequence {
              tunnel: w18 -> [w23]
              tunnel: [w22] -> w15
              tunnel: w14 -> [w21]
              tunnel: [w20] -> w12
              tunnel: w11 -> [w19]
              tunnel: [w57] -> w17
              tunnel: [w56] -> w16
              tunnel: w15 -> [w53]
              tunnel: [w52] -> w13
              tunnel: w12 -> [w52]
              frame #0 {
                n5 = case shown="真" w21 {
                  tunnel: w23 -> [w25 w35]
                  tunnel: [w25 w34] -> w22
                  tunnel: [w24 w30] -> w20
                  tunnel: w19 -> [w24 w26]
                  frame False {
                  }
                  frame True {
                    n6 = flat-sequence {
                      tunnel: w35 -> [w39]
                      tunnel: [w37] -> w33
                      tunnel: [w36] -> w27
                      tunnel: w26 -> [w36]
                      tunnel: w33 -> [w43]
                      tunnel: [w41] -> w32
                      tunnel: [w40] -> w28
                      tunnel: w27 -> [w40]
                      tunnel: w32 -> [w47]
                      tunnel: [w45] -> w31
                      tunnel: [w44] -> w29
                      tunnel: w28 -> [w44]
                      tunnel: [w49] -> w34
                      tunnel: w31 -> [w51]
                      tunnel: [w48] -> w30
                      tunnel: w29 -> [w48]
                      frame #0 {
                        n7 = shared-variable "我的电脑\\Input.lvlib\\Temp_Start_LT"(error in=w39) -> (w38:dbl, error out=w37:errorcluster)
                        n8 = local write "开始温度"(w38) -> ()
                      }
                      frame #1 {
                        n9 = shared-variable "我的电脑\\Input.lvlib\\Temp_Rate_LT"(error in=w43) -> (w42:dbl, error out=w41:errorcluster)
                        n10 = local write "变温速率"(w42) -> ()
                      }
                      frame #2 {
                        n11 = shared-variable "我的电脑\\Input.lvlib\\Temp_End_LT"(error in=w47) -> (w46:dbl, error out=w45:errorcluster)
                        n12 = local write "结束温度"(w46) -> ()
                      }
                      frame #3 {
                        n13 = shared-variable "我的电脑\\Input.lvlib\\Freq_LT"(error in=w51) -> (w50:dbl, error out=w49:errorcluster)
                        n14 = local write "测试频率2"(w50) -> ()
                      }
                    }
                  }
                }
              }
              frame #1 {
                n15 = shared-variable "我的电脑\\Input.lvlib\\Start_LT"(error in=w53) -> (w54:bool, error out=w57:errorcluster)
                n16 = Or(x="低温", y=w54) -> (x .or. y?=w56:bool)
              }
            }
          }
        }
        frame "常温介电测试" {
          n17 = while {
            tunnel: [w63] -> w61
            tunnel: w60 -> [w63]
            tunnel: [w62] -> w58
            tunnel: w59 -> [w62]
            stop <- "开始测量" stop-if-true
          }
        }
        frame "介电偏压测试" {
          n18 = while {
            tunnel: w69 -> [w77]
            tunnel: w68 -> [w76]
            tunnel: [w75] -> w67
            tunnel: w66 -> [w72]
            tunnel: [w70] -> w65
            stop <- w74 stop-if-true
            n19 = flat-sequence {
              tunnel: w77 -> [w82]
              tunnel: w76 -> [w81]
              tunnel: [w80] -> w73
              tunnel: w72 -> [w79]
              tunnel: [w78] -> w71
              tunnel: [w172] -> w75
              tunnel: [w169] -> w74
              tunnel: w73 -> [w168]
              tunnel: [w167] -> w70
              tunnel: w71 -> [w167]
              frame #0 {
                n20 = case shown="假" w81 {
                  tunnel: w82 -> [w84 w88]
                  tunnel: [w84 w87] -> w80
                  tunnel: w79 -> [w83 w86]
                  tunnel: [w83 w85] -> w78
                  frame False {
                  }
                  frame True {
                    n21 = stacked-sequence {
                      seq-local: [w96 _ _ _] -> [_ w120 _ _]
                      seq-local: [w91 _ _ _] -> [_ w114 _ _]
                      seq-local: [w90 _ _ _] -> [_ w113 _ _]
                      seq-local: [_ w119 _ _] -> [_ _ w145 _]
                      seq-local: [_ w115 _ _] -> [_ _ w139 _]
                      seq-local: [_ w114 _ _] -> [_ _ w138 _]
                      seq-local: [_ w112 _ _] -> [_ _ w136 _]
                      seq-local: [_ _ w144 _] -> [_ _ _ w162]
                      seq-local: [_ _ w143 _] -> [_ _ _ w163]
                      seq-local: [_ _ w139 _] -> [_ _ _ w164]
                      seq-local: [_ _ w138 _] -> [_ _ _ w165]
                      seq-local: [_ _ w137 _] -> [_ _ _ w161]
                      tunnel: w88 -> [w95 _ _ _]
                      tunnel: w86 -> [w89 _ _ _]
                      tunnel: [_ _ _ w162] -> w87
                      tunnel: [_ _ _ w161] -> w85
                      frame #0 {
                        n22 = stacked-sequence {
                          seq-local: [w100 _ _] -> [_ w105 _]
                          seq-local: [w98 _ _] -> [_ w102 _]
                          seq-local: [w97 _ _] -> [_ w101 _]
                          seq-local: [_ w104 _] -> [_ _ w111]
                          seq-local: [_ w102 _] -> [_ _ w108]
                          seq-local: [_ w103 _] -> [_ _ w107]
                          seq-local: [_ w101 _] -> [_ _ w106]
                          tunnel: w95 -> [w99 _ _]
                          tunnel: w89 -> [w97 _ _]
                          tunnel: [_ _ w110] -> w96
                          tunnel: [_ _ w108] -> w94
                          tunnel: [_ _ w107] -> w93
                          tunnel: [_ _ w109] -> w92
                          tunnel: [_ _ w106] -> w90
                          frame #0 {
                            n23 = shared-variable "我的电脑\\Input.lvlib\\Phase_1_Volt_Start"(error in=w99) -> (w98:dbl, error out=w100:errorcluster)
                          }
                          frame #1 {
                            n24 = shared-variable "我的电脑\\Input.lvlib\\Phase_1_Volt_End"(error in=w105) -> (w103:dbl, error out=w104:errorcluster)
                          }
                          frame #2 {
                            n25 = shared-variable "我的电脑\\Input.lvlib\\Phase_1_Volt_Step"(error in=w111) -> (w109:dbl, error out=w110:errorcluster)
                          }
                        }
                        n26 = Build Array(w94, w93, w92) -> (w91:dbl[])
                      }
                      frame #1 {
                        n27 = stacked-sequence {
                          seq-local: [w123 _ _] -> [_ w129 _]
                          seq-local: [w122 _ _] -> [_ w126 _]
                          seq-local: [w121 _ _] -> [_ w125 _]
                          seq-local: [_ w128 _] -> [_ _ w135]
                          seq-local: [_ w127 _] -> [_ _ w132]
                          seq-local: [_ w126 _] -> [_ _ w131]
                          seq-local: [_ w125 _] -> [_ _ w130]
                          tunnel: w120 -> [w124 _ _]
                          tunnel: w113 -> [w121 _ _]
                          tunnel: [_ _ w134] -> w119
                          tunnel: [_ _ w133] -> w118
                          tunnel: [_ _ w132] -> w117
                          tunnel: [_ _ w131] -> w116
                          tunnel: [_ _ w130] -> w112
                          frame #0 {
                            n28 = shared-variable "我的电脑\\Input.lvlib\\Phase_2_Volt_Start"(error in=w124) -> (w122:dbl, error out=w123:errorcluster)
                          }
                          frame #1 {
                            n29 = shared-variable "我的电脑\\Input.lvlib\\Phase_2_Volt_End"(error in=w129) -> (w127:dbl, error out=w128:errorcluster)
                          }
                          frame #2 {
                            n30 = shared-variable "我的电脑\\Input.lvlib\\Phase_2_Volt_Step"(error in=w135) -> (w133:dbl, error out=w134:errorcluster)
                          }
                        }
                        n31 = Build Array(w116, w117, w118) -> (w115:dbl[])
                      }
                      frame #2 {
                        n32 = stacked-sequence {
                          seq-local: [w148 _ _] -> [_ w154 _]
                          seq-local: [w147 _ _] -> [_ w151 _]
                          seq-local: [w146 _ _] -> [_ w150 _]
                          seq-local: [_ w153 _] -> [_ _ w160]
                          seq-local: [_ w152 _] -> [_ _ w157]
                          seq-local: [_ w151 _] -> [_ _ w156]
                          seq-local: [_ w150 _] -> [_ _ w155]
                          tunnel: w145 -> [w149 _ _]
                          tunnel: w136 -> [w146 _ _]
                          tunnel: [_ _ w159] -> w144
                          tunnel: [_ _ w158] -> w142
                          tunnel: [_ _ w157] -> w141
                          tunnel: [_ _ w156] -> w140
                          tunnel: [_ _ w155] -> w137
                          frame #0 {
                            n33 = shared-variable "我的电脑\\Input.lvlib\\Phase_3_Volt_Start"(error in=w149) -> (w147:dbl, error out=w148:errorcluster)
                          }
                          frame #1 {
                            n34 = shared-variable "我的电脑\\Input.lvlib\\Phase_3_Volt_End"(error in=w154) -> (w152:dbl, error out=w153:errorcluster)
                          }
                          frame #2 {
                            n35 = shared-variable "我的电脑\\Input.lvlib\\Phase_3_Volt_Step"(error in=w160) -> (w158:dbl, error out=w159:errorcluster)
                          }
                        }
                        n36 = Build Array(w140, w141, w142) -> (w143:dbl[])
                      }
                      frame #3 {
                        n37 = Build Array(w165, w164, w163) -> (w166:dbl[][])
                        n38 = local write "起始偏压"(w166) -> ()
                      }
                    }
                  }
                }
              }
              frame #1 {
                n39 = shared-variable "我的电脑\\Input.lvlib\\Start_BI"(error in=w168) -> (w170:bool, error out=w172:errorcluster)
                n40 = Or(x=w170, y="偏压") -> (x .or. y?=w169:bool)
              }
            }
          }
        }
        frame "介电频谱测试" {
          n41 = while {
            tunnel: w177 -> [w185]
            tunnel: w176 -> [w184]
            tunnel: [w183] -> w175
            tunnel: [w180] -> w174
            tunnel: w173 -> [w178]
            stop <- w182 stop-if-true
            n42 = flat-sequence {
              tunnel: w185 -> [w190]
              tunnel: w184 -> [w189]
              tunnel: [w188] -> w181
              tunnel: [w187] -> w179
              tunnel: w178 -> [w186]
              tunnel: [w244] -> w183
              tunnel: [w241] -> w182
              tunnel: w181 -> [w240]
              tunnel: [w239] -> w180
              tunnel: w179 -> [w239]
              frame #0 {
                n43 = case shown="真" w189 {
                  tunnel: w190 -> [w192 w200]
                  tunnel: [w192 w199] -> w188
                  tunnel: [w191 w193] -> w187
                  tunnel: w186 -> [w191 w194]
                  frame False {
                  }
                  frame True {
                    n44 = flat-sequence {
                      tunnel: w200 -> [w214]
                      tunnel: [w215] -> w198
                      tunnel: [w204] -> w195
                      tunnel: w194 -> [w201]
                      tunnel: w198 -> [w233]
                      tunnel: [w234] -> w197
                      tunnel: [w231] -> w196
                      tunnel: w195 -> [w231]
                      tunnel: [w236] -> w199
                      tunnel: w197 -> [w237]
                      tunnel: w196 -> [w235]
                      tunnel: [w235] -> w193
                      frame #0 {
                        n45 = flat-sequence {
                          tunnel: w214 -> [w218]
                          tunnel: [w219] -> w209
                          tunnel: [w217] -> w208
                          tunnel: [w216] -> w202
                          tunnel: w201 -> [w216]
                          tunnel: w209 -> [w223]
                          tunnel: w208 -> [w221]
                          tunnel: [w224] -> w207
                          tunnel: [w221] -> w206
                          tunnel: [w222] -> w205
                          tunnel: [w220] -> w203
                          tunnel: w202 -> [w220]
                          tunnel: [w230] -> w215
                          tunnel: [w227] -> w212
                          tunnel: [w226] -> w211
                          tunnel: [w228] -> w210
                          tunnel: w207 -> [w229]
                          tunnel: w206 -> [w227]
                          tunnel: w205 -> [w226]
                          tunnel: [w225] -> w204
                          tunnel: w203 -> [w225]
                          frame #0 {
                            n46 = shared-variable "我的电脑\\Input.lvlib\\Freq_Start"(error in=w218) -> (w217:dbl, error out=w219:errorcluster)
                          }
                          frame #1 {
                            n47 = shared-variable "我的电脑\\Input.lvlib\\Freq_End"(error in=w223) -> (w222:dbl, error out=w224:errorcluster)
                          }
                          frame #2 {
                            n48 = shared-variable "我的电脑\\Input.lvlib\\Freq_Step"(error in=w229) -> (w228:dbl, error out=w230:errorcluster)
                          }
                        }
                        n49 = Build Array(w212, w211, w210) -> (w213:dbl[])
                        n50 = local write "开始频率"(w213) -> ()
                      }
                      frame #1 {
                        n51 = shared-variable "我的电脑\\Input.lvlib\\Time_Span"(error in=w233) -> (w232:dbl, error out=w234:errorcluster)
                        n52 = local write "时间间隔(s)"(w232) -> ()
                      }
                      frame #2 {
                        n53 = shared-variable "我的电脑\\Input.lvlib\\Scan_Mode"(error in=w237) -> (w238:i16, error out=w236:errorcluster)
                        n54 = local write "Scanning Mode"(w238) -> ()
                      }
                    }
                  }
                }
              }
              frame #1 {
                n55 = shared-variable "我的电脑\\Input.lvlib\\Start_SP"(error in=w240) -> (w243:bool, error out=w244:errorcluster)
                n56 = Or(x="频谱", y=w243) -> (x .or. y?=w241:bool)
              }
            }
          }
        }
        frame "常温绝缘测试" {
          n57 = while {
            tunnel: w249 -> [w257]
            tunnel: w248 -> [w256]
            tunnel: [w255] -> w247
            tunnel: w246 -> [w252]
            tunnel: [w250] -> w245
            stop <- w254 stop-if-true
            n58 = flat-sequence {
              tunnel: w257 -> [w262]
              tunnel: w256 -> [w261]
              tunnel: [w260] -> w253
              tunnel: w252 -> [w259]
              tunnel: [w258] -> w251
              tunnel: [w296] -> w255
              tunnel: [w293] -> w254
              tunnel: w253 -> [w292]
              tunnel: [w291] -> _
              tunnel: w251 -> [w291]
              tunnel: [w291] -> w250
              frame #0 {
                n59 = case shown="假" w261 {
                  tunnel: w262 -> [w264 w273]
                  tunnel: [w264 w274] -> w260
                  tunnel: [w263 w269] -> w258
                  tunnel: w259 -> [w263 w265]
                  frame False {
                  }
                  frame True {
                    n60 = flat-sequence {
                      tunnel: w273 -> [w276]
                      tunnel: [w278] -> w272
                      tunnel: [w275] -> w266
                      tunnel: w265 -> [w275]
                      tunnel: w272 -> [w282]
                      tunnel: [w281] -> w271
                      tunnel: [w279] -> w267
                      tunnel: w266 -> [w279]
                      tunnel: w271 -> [w286]
                      tunnel: [w285] -> w270
                      tunnel: [w283] -> w268
                      tunnel: w267 -> [w283]
                      tunnel: [w289] -> w274
                      tunnel: w270 -> [w290]
                      tunnel: [w287] -> w269
                      tunnel: w268 -> [w287]
                      frame #0 {
                        n61 = shared-variable "我的电脑\\Input.lvlib\\Time_IN"(error in=w276) -> (w277:dbl, error out=w278:errorcluster)
                        n62 = local write "测试时间"(w277) -> ()
                      }
                      frame #1 {
                        n63 = shared-variable "我的电脑\\Input.lvlib\\Volt_IN"(error in=w282) -> (w280:dbl, error out=w281:errorcluster)
                        n64 = local write "电压(V)"(w280) -> ()
                      }
                      frame #2 {
                        n65 = shared-variable "我的电脑\\Input.lvlib\\Sample_Diameter"(error in=w286) -> (w284:dbl, error out=w285:errorcluster)
                        n66 = local write "样本直径(mm)"(w284) -> ()
                      }
                      frame #3 {
                        n67 = shared-variable "我的电脑\\Input.lvlib\\Sample_Thickness"(error in=w290) -> (w288:dbl, error out=w289:errorcluster)
                        n68 = local write "样本厚度(mm)"(w288) -> ()
                      }
                    }
                  }
                }
              }
              frame #1 {
                n69 = shared-variable "我的电脑\\Input.lvlib\\Start_IN"(error in=w292) -> (w294:bool, error out=w296:errorcluster)
                n70 = Or(x=w294, y="绝缘") -> (x .or. y?=w293:bool)
              }
            }
          }
        }
        frame "Cole-Cole图" {
          n71 = while {
            tunnel: [w302] -> w299
            tunnel: w300 -> [w302]
            tunnel: [w301] -> w297
            tunnel: w298 -> [w301]
            stop <- "开始测量" stop-if-true
          }
        }
        frame "热激励极化电流" {
          n72 = while {
            tunnel: [w310] -> w306
            tunnel: w307 -> [w310]
            tunnel: [w308] -> w304
            tunnel: w305 -> [w308]
            stop <- "极化开始" stop-if-true
          }
        }
        frame "温度设置".. {
          n73 = while {
            tunnel: w315 -> [w323]
            tunnel: w314 -> [w322]
            tunnel: [w320] -> w313
            tunnel: w312 -> [w318]
            tunnel: [w316] -> w311
            stop <- w319 stop-if-true
            n74 = flat-sequence {
              tunnel: w323 -> [w328]
              tunnel: w322 -> [w327]
              tunnel: [w326] -> w321
              tunnel: w318 -> [w325]
              tunnel: [w324] -> w317
              tunnel: w321 -> [w350]
              tunnel: [w349] -> w320
              tunnel: [w346] -> w319
              tunnel: w317 -> [w345]
              tunnel: [w345] -> w316
              frame #0 {
                n75 = case shown="假" w327 {
                  tunnel: w328 -> [w330 w336]
                  tunnel: [w330 w335] -> w326
                  tunnel: w325 -> [w329 w332]
                  tunnel: [w329 w331] -> w324
                  frame False {
                  }
                  frame True {
                    n76 = flat-sequence {
                      tunnel: w336 -> [w338]
                      tunnel: [w340] -> w334
                      tunnel: [w337] -> w333
                      tunnel: w332 -> [w337]
                      tunnel: [w343] -> w335
                      tunnel: w334 -> [w344]
                      tunnel: [w341] -> w331
                      tunnel: w333 -> [w341]
                      frame #0 {
                        n77 = shared-variable "我的电脑\\Input.lvlib\\Temp_TE"(error in=w338) -> (w339:dbl, error out=w340:errorcluster)
                        n78 = local write "目标温度"(w339) -> ()
                      }
                      frame #1 {
                        n79 = shared-variable "我的电脑\\Input.lvlib\\Rate_TE"(error in=w344) -> (w342:dbl, error out=w343:errorcluster)
                        n80 = local write "变温速率1"(w342) -> ()
                      }
                    }
                  }
                }
              }
              frame #1 {
                n81 = shared-variable "我的电脑\\Input.lvlib\\Start_TE"(error in=w350) -> (w347:bool, error out=w349:errorcluster)
                n82 = Or(x=w347, y="温度") -> (x .or. y?=w346:bool)
              }
            }
          }
        }
      }
    }
    frame #1 {
      n83 = case shown="\"Cole-Cole图\"" w351 {
        selector: w351 -> [w368 _ _ _ _ _ _ _]
        tunnel: [w383 w419 w425 w432 w453 w470 w487 w493] -> w352
        tunnel: w353 -> [w367 w418 w426 w433 w454 w469 w488 w494]
        frame .."变温介电测试 ", Default {
          n84 = local read "CT_LT"() -> (w372:cluster{dbl[], dbl[]})
          n85 = local read "LT_LT"() -> (w371:cluster{dbl[], dbl[]})
          n86 = Bundle("测试频率1"="测试频率1", "测试频率2"="测试频率2", "测试频率3"="测试频率3", "测试频率4"="测试频率4") -> (w355:T2)  [unwired: 1 in]
          n87 = Bundle("CT_LT"=w372, "LT_LT"=w371) -> (w373:T3)  [unwired: 1 in]
          n88 = Less Or Equal?(x="结束温度", y=250) -> (x <= y?=w364:bool)
          n89 = Bundle("电容计地址"="电容计地址", "高温地址 1"="高温地址 1", "高温地址 2"="高温地址 2") -> (w360:T4)  [unwired: 1 in]
          n90 = Bundle("表格（L）路径："="表格（L）路径：", "文本（L）路径："="文本（L）路径：") -> (w377:cluster{"表格（L）路径：":path, "文本（L）路径：":path})  [unwired: 1 in]
          n91 = Bundle("开始温度"="开始温度", "变温速率"="变温速率", "结束温度"="结束温度", w355) -> (w376:T5)  [unwired: 1 in]
          n92 = Bundle("电容计地址"="电容计地址", "低温地址"="低温地址") -> (w375:T6)  [unwired: 1 in]
          n93 = case shown="真" "低温 2" {
            tunnel: w373 -> [_ w405]
            tunnel: w368 -> [_ w404]
            frame False {
            }
            frame True {
              n94 = call "DP.vi"("Cluster 2"=w405, "Boolean"="TCC趋势", "Ring 2"="LT拟合", "Ring"="CT拟合", "Numeric"=w404) -> ("XY Graph 2"=→"LT_LT":cluster{dbl[], "Best Gaussian Fit":dbl[]}, "XY Graph"=→"CT_LT":cluster{dbl[], "Array":dbl[]}, "RES_LT"=→"残差（损耗）":dbl, "RES_CT"=→"残差（电容）":dbl, "TCC"=→"TCC(ppm/℃)":dbl)  [unwired: 2 in]
            }
          }
          n95 = control-ref of="CT_LT"() -> (w370:refnum<vi>)
          n96 = control-ref of="LT_LT"() -> (w369:refnum<vi>)
          n97 = case shown="假" w364 {
            tunnel: [w387 w399] -> w383
            tunnel: w377 -> [w391 w398]
            tunnel: w376 -> [w390 w397]
            tunnel: w375 -> [_ w396]
            tunnel: w370 -> [w386 w395]
            tunnel: w369 -> [w385 w394]
            tunnel: w367 -> [w388 w393]
            tunnel: w360 -> [w389 _]
            tunnel: "功能选择" -> [w384 w392]
            frame False {
              n98 = call "HT.vi"("Ctl Refnum 2"=w385, "Ctl Refnum"=w386, "Function (0: Cp-D)"=w384, "error in (no error)"=w388, "Cluster"=w389, "Cluster 2"=w390, "Cluster 3"=w391) -> ("错误输出"=w387:cluster{"状态":bool, "代码":i32, "源":string})  [unwired: 4 in]
            }
            frame True {
              n99 = call "LT.vi"("Ctl Refnum 2"=w394, "Ctl Refnum"=w395, "Function (0: Cp-D)"=w392, "error in (no error)"=w393, "Cluster 3"=w396, "Cluster"=w397, "Cluster 2"=w398) -> ("错误输出"=w399:cluster{"状态":bool, "代码":i32, "源":string})  [unwired: 4 in]
            }
          }
        }
        frame "常温介电测试" {
          n100 = Bundle("文本（R）路径："="文本（R）路径：", "表格（R）路径："="表格（R）路径：") -> (w413:cluster{"文本（R）路径：":path, "表格（R）路径：":path})  [unwired: 1 in]
          n101 = local read "电容计地址"() -> (w411:refnum<visa-resource-name>)
          n102 = control-ref of="LT_RT"() -> (w416:refnum<vi>)
          n103 = control-ref of="CT_RT"() -> (w417:refnum<vi>)
          n104 = call "CT.vi"("Ctl Refnum 2"=w416, "Ctl Refnum"=w417, "测试时长"="测试时长（s）", "error in (no error)"=w418, "客户仪器地址"=w411, "测试频率"="测试频率（Hz）", "Cluster 2"=w413) -> ("错误输出"=w419:cluster{"状态":bool, "代码":i32, "源":string})  [unwired: 4 in]
        }
        frame "介电偏压测试" {
          n105 = Bundle("表格（BI）路径："="表格（BI）路径：", "文本（BI）路径："="文本（BI）路径：") -> (w422:cluster{"表格（BI）路径：":path, "文本（BI）路径：":path})  [unwired: 1 in]
          n106 = local read "电容计地址"() -> (w428:refnum<visa-resource-name>)
          n107 = control-ref of="?"() -> (w420:refnum<vi>)
          n108 = control-ref of="?"() -> (w421:refnum<vi>)
          n109 = call "BI.vi"("Ctl Refnum 2"=w420, "Ctl Refnum"=w421, "error in (no error)"=w426, "客户仪器地址"=w428, "Cluster 2"=w422, "起始偏压"="起始偏压") -> ("错误输出"=w425:cluster{"状态":bool, "代码":i32, "源":string})  [unwired: 5 in]
        }
        frame "介电频谱测试" {
          n110 = local read "电容计地址"() -> (w436:refnum<visa-resource-name>)
          n111 = control-ref of="?"() -> (w429:refnum<vi>)
          n112 = control-ref of="?"() -> (w430:refnum<vi>)
          n113 = call "SP.vi"("Ctl Refnum 2"=w429, "Ctl Refnum"=w430, "表格（SP）路径："="表格（SP）路径：", "时间间隔(s)"="时间间隔(s)", "开始频率"="开始频率", "error in (no error)"=w433, "客户仪器地址"=w436, "Scanning Mode"="Scanning Mode", "文本（SP）路径："="文本（SP）路径：") -> ("错误输出"=w432:cluster{"状态":bool, "代码":i32, "源":string})  [unwired: 2 in]
        }
        frame "常温绝缘测试" {
          n114 = local read "电容计地址"() -> (w449:refnum<visa-resource-name>)
          n115 = local read "高温地址 2"() -> (w451:refnum<visa-resource-name>)
          n116 = local read "低温地址"() -> (w452:refnum<visa-resource-name>)
          n117 = Bundle("电阻计地址"="电阻计地址", "电容计地址"=w449, "低温地址"=w452, "高温地址 2"=w451) -> (w450:T7)  [unwired: 1 in]
          n118 = Bundle("电压(V)"="电压(V)", "样本直径(mm)"="样本直径(mm)", "样本厚度(mm)"="样本厚度(mm)") -> (w447:T8)  [unwired: 1 in]
          n119 = control-ref of="?"() -> (w445:refnum<vi>)
          n120 = control-ref of="?"() -> (w446:refnum<vi>)
          n121 = call "IN.vi"("Ctl Refnum 2"=w445, "Ctl Refnum"=w446, "Cluster 3"=w447, "6517B"="使用6517B", "测试时间"="测试时间", "error in (no error)"=w454, "Cluster"=w450, "文本"="文本（IN）路径：", "表格"="表格（IN）路径：") -> ("错误输出"=w453:cluster{"状态":bool, "代码":i32, "源":string})  [unwired: 2 in]
        }
        frame "Cole-Cole图" {
          n122 = local read "电容计地址"() -> (w459:refnum<visa-resource-name>)
          n123 = local read "高温地址 1"() -> (w458:refnum<visa-resource-name>)
          n124 = local read "高温地址 2"() -> (w457:refnum<visa-resource-name>)
          n125 = control-ref of="当前频率"() -> (w464:refnum<vi>)
          n126 = control-ref of="炉丝温度"() -> (w463:refnum<vi>)
          n127 = control-ref of="设定温度"() -> (w462:refnum<vi>)
          n128 = control-ref of="样品温度"() -> (w461:refnum<vi>)
          n129 = control-ref of="?"() -> (w465:refnum<vi>)
          n130 = Bundle("电容计地址"=w459, "高温地址 1"=w458, "高温地址 2"=w457) -> (w456:T4)  [unwired: 1 in]
          n131 = Bundle("Ctrl Reference"=w465, "当前频率"=w464, "炉丝温度"=w463, "设定温度"=w462, "样品温度"=w461) -> (w460:T9)  [unwired: 1 in]
          n132 = call "CC.vi"("测试温度"="测试温度", "簇 2"=w460, "Scanning Mode"="扫描模式", "开始频率"="开始频率", "error in (no error)"=w469, "簇"=w456, "文本"="文本（CC）路径：", "表格"="表格（CC）路径：") -> ("错误输出"=w470:cluster{"状态":bool, "代码":i32, "源":string})  [unwired: 3 in]
        }
        frame "热激励极化电流" {
          n133 = local read "电阻计地址"() -> (w492:refnum<visa-resource-name>)
          n134 = local read "高温地址 1"() -> (w491:refnum<visa-resource-name>)
          n135 = local read "高温地址 2"() -> (w490:refnum<visa-resource-name>)
          n136 = Bundle("电阻计地址"=w492, "高温地址 1"=w491, "高温地址 2"=w490) -> (w489:T10)  [unwired: 1 in]
          n137 = Bundle("变温速率（℃/min）"="变温速率（℃/min）", "极化温度（℃）"="极化温度（℃）", "极化电压（V）"="极化电压（V）", "极化时间"="极化时间") -> (w482:T11)  [unwired: 1 in]
          n138 = control-ref of="?"() -> (w481:refnum<vi>)
          n139 = call "DC.vi"("结束冷却"="结束冷却", "文本（TSDC）路径："="文本（TSDC）路径：", "Ctl Refnum"=w481, "error in (no error)"=w488, "结束温度"="结束温度（℃）", "簇 2"=w482, "簇"=w489) -> ("error out"=w487:errorcluster, "极化电流"=→"当前去极化电流":dbl, "簇 3"=w477:cluster{"当前温度":dbl, "当前电压":bool, "剩余时间":dbl})  [unwired: 2 in]
          n140 = Unbundle(w477) -> ("当前温度"=→"当前温度":dbl, "当前电压"=→"极化状态":bool, "剩余时间"=→"剩余时间":dbl)
        }
        frame "温度设置".. {
          n141 = local read "高温地址 2"() -> (w496:refnum<visa-resource-name>)
          n142 = local read "高温地址 1"() -> (w497:refnum<visa-resource-name>)
          n143 = local read "低温地址"() -> (w498:refnum<visa-resource-name>)
          n144 = control-ref of="TE"() -> (w495:refnum<vi>)
          n145 = call "TE.vi"("Ctl Refnum"=w495, "error in (no error)"=w494, "目标温度"="目标温度", "低温地址"=w498, "高温"=w497, "高温 2"=w496, "变温速率1"="变温速率1") -> ("error out"=w493:errorcluster)  [unwired: 4 in]
        }
      }
      "错误输出" <- w352
    }
  }
